vi "Read page name, size and orientation from PDF file.vi"(0 "PageSizeWithRotation":refnum<k24>, 11 "error in (no error)":errorcluster) -> (4 "PageSizeWithRotation duplicate":refnum<k24>, 8 "Pages dimensions OUT":T1={"Start at page"=-1, "Page Size"=0, "Orientation"=enum."Portrait", "widht"=0.0, "height"=0.0, "Margin left"=0.0, "Margin right"=0.0, "Margin top"=0.0, "Margin bottom"=0.0, "X0"=0.0, "X1"=612.0, "Y0"=0.0, "Y1"=792.0} {"Page Size" items=["Custom", "LETTER", "NOTE", "LEGAL", "TABLOID", "EXECUTIVE", "POSTCARD", "A0", "A1", "A2", "A3", "A4", "A5", "A6", "A7", "A8", "A9", "A10", "B0", "B1", "B2", "B3", "B4", "B5", "B6", "B7", "B8", "B9", "B10", "ARCH_E", "ARCH_D", "ARCH_C", "ARCH_B", "ARCH_A", "FLSA", "FLSE", "HALFLETTER", "_11X17", "ID_1", "ID_2", "ID_3", "LEDGER", "CROWN_QUARTO", "LARGE_CROWN_QUARTO", "DEMY_QUARTO", "ROYAL_QUARTO", "CROWN_OCTAVO", "LARGE_CROWN_OCTAVO", "DEMY_OCTAVO", "ROYAL_OCTAVO", "SMALL_PAPERBACK", "PENGUIN_SMALL_PAPERBACK", "PENGUIN_LARGE_PAPERBACK"]}, 15 "error out":errorcluster)   [LabVIEW 2019, in "Exaprom PDF.lvlib"]
doc: "Version 1.1\nDeveloped by Jean-Marc Simard\nCopyright © 2012, Exaprom Inc.\nAll rights reserved.\nLicense: BSD\n\nWith iTextSharp 4.1.6 (http://itextsharp.sourceforge.net)\nunder Mozilla Public License Version 1.1\n(http://www.mozilla.org/MPL/MPL-1.1.html)"
uses:
  C:/work/niobrara_lv/labview pdf writer fixing/DLL/itextsharp.dll
  DLL/itextsharp.dll
  Controls/Page Controls/Page dimensions.ctl
  Controls/Page Controls/Page Orientation.ctl
  Exaprom PDF.lvlib
  Controls/Page Controls/Page size.ctl
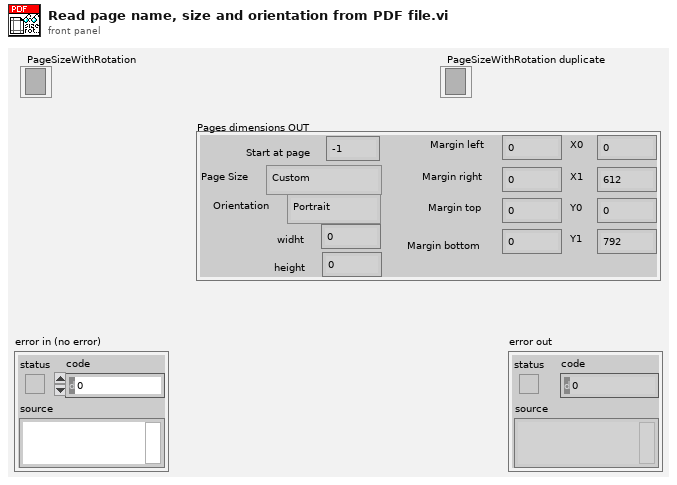
[diagram p1: front panel]
types:
  T1 = typedef "Exaprom PDF.lvlib/Page dimensions.ctl" = cluster{"Start at page":i32, "Page Size":T2, "Orientation":T3, "widht":sgl, "height":sgl, "Margin left":sgl, "Margin right":sgl, "Margin top":sgl, "Margin bottom":sgl, "X0":sgl, "X1":sgl, "Y0":sgl, "Y1":sgl}
  T2 = typedef "Exaprom PDF.lvlib/Page size.ctl" = i32
  T3 = typedef "Exaprom PDF.lvlib/Page Orientation.ctl" = enum16{"Portrait", "Landscape"}
  T4 = cluster{"Name":string, "Width":sgl, "Height":sgl}[]
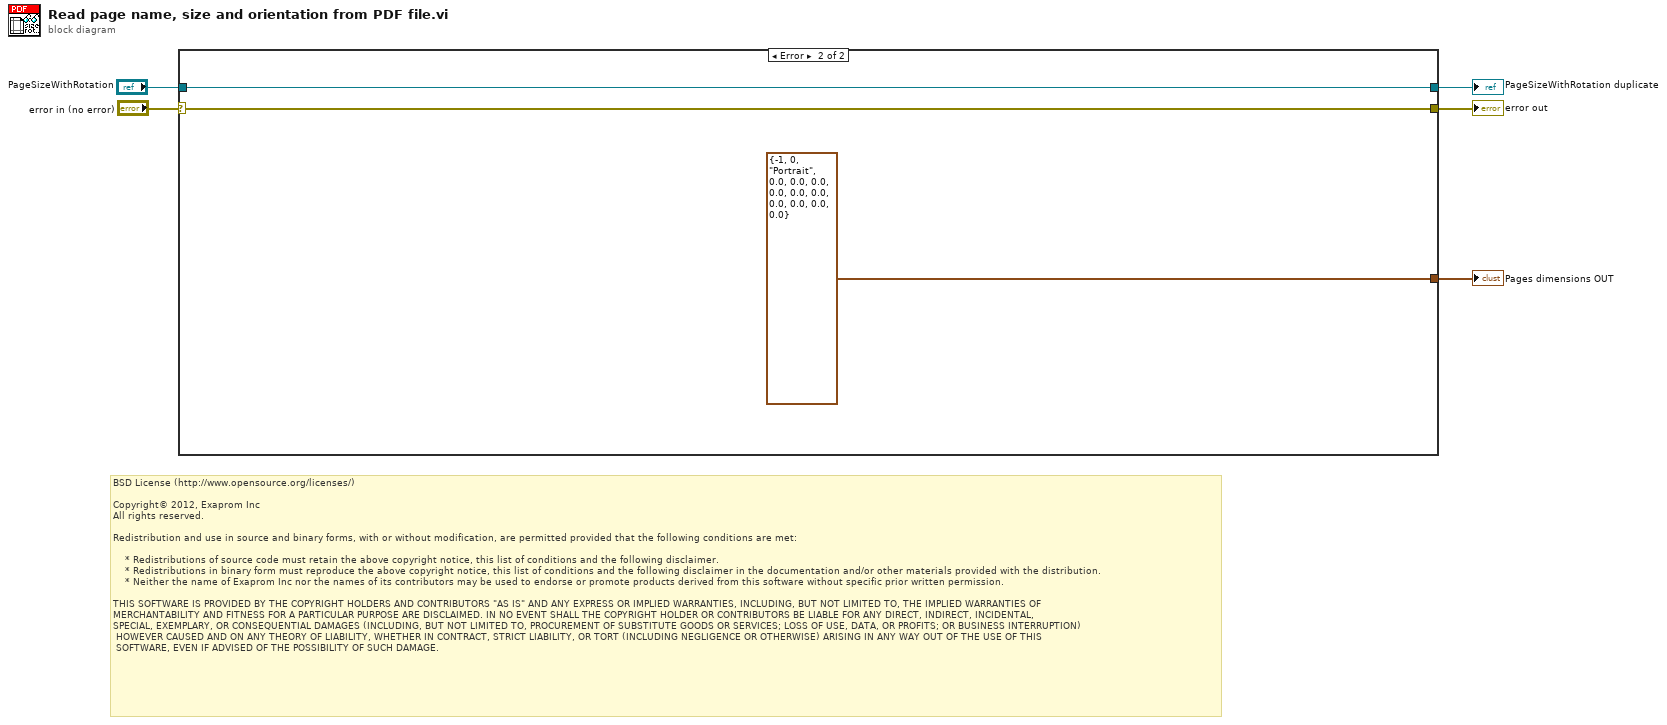
[diagram p0: block diagram]
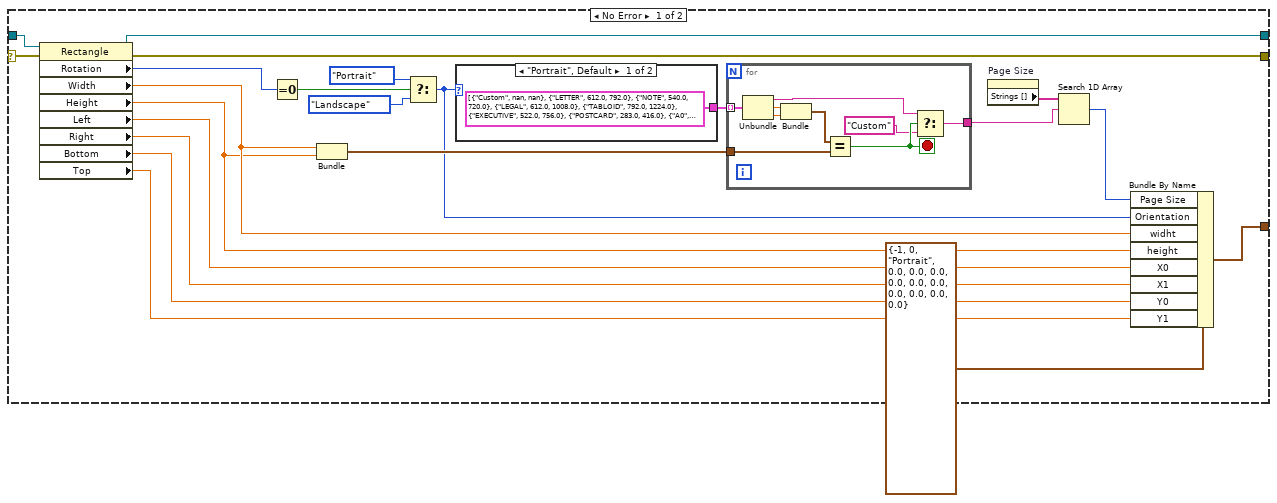
[diagram p2: hidden frame]
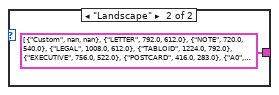
[diagram p3: hidden frame]
diagram:
  # "BSD License (http://www.opensource.org/licenses/)\n\nCopyright© 2012, Exaprom Inc\nAll rights reserved.\n\nRedistribution and use in source and binary forms, with or without modification, are permitted provided that the following conditions are met:\n\n    * Redistributions of source code must retain the above copyright notice, this list of conditions and the following disclaimer.\n    * Redistributions in binary form must reproduce the above copyright notice, this list of conditions and the following disclaimer in the documentation and/or other materials provided with the distribution.\n    * Neither the name of Exaprom Inc nor the names of its contributors may be used to endorse or promote products derived from this software without specific prior written permission.\n\nTHIS SOFTWARE IS PROVIDED BY THE COPYRIGHT HOLDERS AND CONTRIBUTORS \"AS IS\" AND ANY EXPRESS OR IMPLIED WARRANTIES, INCLUDING, BUT NOT LIMITED TO, THE IMPLIED WARRANTIES OF \nMERCHANTABILITY AND FITNESS FOR A PARTICULAR PURPOSE ARE DISCLAIMED. IN NO EVENT SHALL THE COPYRIGHT HOLDER OR CONTRIBUTORS BE LIABLE FOR ANY DIRECT, INDIRECT, INCIDENTAL,\nSPECIAL, EXEMPLARY, OR CONSEQUENTIAL DAMAGES (INCLUDING, BUT NOT LIMITED TO, PROCUREMENT OF SUBSTITUTE GOODS OR SERVICES; LOSS OF USE, DATA, OR PROFITS; OR BUSINESS INTERRUPTION)\n HOWEVER CAUSED AND ON ANY THEORY OF LIABILITY, WHETHER IN CONTRACT, STRICT LIABILITY, OR TORT (INCLUDING NEGLIGENCE OR OTHERWISE) ARISING IN ANY WAY OUT OF THE USE OF THIS\n SOFTWARE, EVEN IF ADVISED OF THE POSSIBILITY OF SUCH DAMAGE."
  n1 = case shown="Error" "error in (no error)" {
    selector: "error in (no error)" -> [w22 w41]
    tunnel: [w23 w41] -> w5
    tunnel: "PageSizeWithRotation" -> [w21 w40]
    tunnel: [w20 w40] -> w2
    tunnel: [w11 T1 {"Start at page"=-1, "Page Size"=0, "Orientation"=enum."Portrait", "widht"=0.0, "height"=0.0, "Margin left"=0.0, "Margin right"=0.0, "Margin top"=0.0, "Margin bottom"=0.0, "X0"=0.0, "X1"=0.0, "Y0"=0.0, "Y1"=0.0} ("output cluster")] -> w1
    frame No Error {
      n2 = property class="Rectangle"(reference=w21, error in=w22) -> (reference out=w20:refnum<k24>, error out=w23:errorcluster, "Rotation"=w27:i32, "Width"=w14:sgl, "Height"=w13:sgl, "Left"=w9:sgl, "Right"=w8:sgl, "Bottom"=w7:sgl, "Top"=w6:sgl)
      n3 = Equal To 0?(x=w27) -> (x = 0?=w26:bool)
      n4 = Bundle("Width"=w14, "Height"=w13) -> (w18:cluster{"Width":sgl, "Height":sgl})  [unwired: 1 in]
      n5 = Select(t=Page_Orientation."Portrait" ("Orientation"), s=w26, f=Page_Orientation."Landscape" ("Orientation")) -> (s? t:f=w15:T3)
      n6 = case shown="\"Portrait\", Default" w15 {
        tunnel: [T4 [{"Name"="Custom", "Width"=nan, "Height"=nan}, {"Name"="LETTER", "Width"=612.0, "Height"=792.0}, {"Name"="NOTE", "Width"=540.0, "Height"=720.0}, {"Name"="LEGAL", "Width"=612.0, "Height"=1008.0}, {"Name"="TABLOID", "Width"=792.0, "Height"=1224.0}, {"Name"="EXECUTIVE", "Width"=522.0, "Height"=756.0}, {"Name"="POSTCARD", "Width"=283.0, "Height"=416.0}, {"Name"="A0", "Width"=2384.0, "Height"=3370.0}, {"Name"="A1", "Width"=1684.0, "Height"=2384.0}, {"Name"="A2", "Width"=1191.0, "Height"=1684.0}, {"Name"="A3", "Width"=842.0, "Height"=1191.0}, {"Name"="A4", "Width"=595.0, "Height"=842.0}, {"Name"="A5", "Width"=420.0, "Height"=595.0}, {"Name"="A6", "Width"=297.0, "Height"=420.0}, {"Name"="A7", "Width"=210.0, "Height"=297.0}, {"Name"="A8", "Width"=148.0, "Height"=210.0}, {"Name"="A9", "Width"=105.0, "Height"=148.0}, {"Name"="A10", "Width"=73.0, "Height"=105.0}, {"Name"="B0", "Width"=2834.0, "Height"=4008.0}, {"Name"="B1", "Width"=2004.0, "Height"=2834.0}, {"Name"="B2", "Width"=1417.0, "Height"=2004.0}, {"Name"="B3", "Width"=1000.0, "Height"=1417.0}, {"Name"="B4", "Width"=708.0, "Height"=1000.0}, {"Name"="B5", "Width"=498.0, "Height"=708.0}, {"Name"="B6", "Width"=354.0, "Height"=498.0}, {"Name"="B7", "Width"=249.0, "Height"=354.0}, {"Name"="B8", "Width"=175.0, "Height"=249.0}, {"Name"="B9", "Width"=124.0, "Height"=175.0}, {"Name"="B10", "Width"=87.0, "Height"=124.0}, {"Name"="ARCH_E", "Width"=2592.0, "Height"=3456.0}, {"Name"="ARCH_D", "Width"=1728.0, "Height"=2592.0}, {"Name"="ARCH_C", "Width"=1296.0, "Height"=1728.0}, {"Name"="ARCH_B", "Width"=864.0, "Height"=1296.0}, {"Name"="ARCH_A", "Width"=648.0, "Height"=864.0}, {"Name"="FLSA", "Width"=612.0, "Height"=936.0}, {"Name"="FLSE", "Width"=648.0, "Height"=936.0}, {"Name"="HALFLETTER", "Width"=396.0, "Height"=612.0}, {"Name"="_11X17", "Width"=792.0, "Height"=1224.0}, {"Name"="ID_1", "Width"=242.65, "Height"=153.0}, {"Name"="ID_2", "Width"=297.0, "Height"=210.0}, {"Name"="ID_3", "Width"=354.0, "Height"=249.0}, {"Name"="LEDGER", "Width"=1224.0, "Height"=792.0}, {"Name"="CROWN_QUARTO", "Width"=535.0, "Height"=697.0}, {"Name"="LARGE_CROWN_QUARTO", "Width"=569.0, "Height"=731.0}, {"Name"="DEMY_QUARTO", "Width"=620.0, "Height"=782.0}, {"Name"="ROYAL_QUARTO", "Width"=671.0, "Height"=884.0}, {"Name"="CROWN_OCTAVO", "Width"=348.0, "Height"=527.0}, {"Name"="LARGE_CROWN_OCTAVO", "Width"=365.0, "Height"=561.0}, {"Name"="DEMY_OCTAVO", "Width"=391.0, "Height"=612.0}, {"Name"="ROYAL_OCTAVO", "Width"=442.0, "Height"=663.0}, {"Name"="SMALL_PAPERBACK", "Width"=314.0, "Height"=504.0}, {"Name"="PENGUIN_SMALL_PAPERBACK", "Width"=314.0, "Height"=513.0}, {"Name"="PENGUIN_LARGE_PAPERBACK", "Width"=365.0, "Height"=561.0}] ("Portrait") T4 [{"Name"="Custom", "Width"=nan, "Height"=nan}, {"Name"="LETTER", "Width"=792.0, "Height"=612.0}, {"Name"="NOTE", "Width"=720.0, "Height"=540.0}, {"Name"="LEGAL", "Width"=1008.0, "Height"=612.0}, {"Name"="TABLOID", "Width"=1224.0, "Height"=792.0}, {"Name"="EXECUTIVE", "Width"=756.0, "Height"=522.0}, {"Name"="POSTCARD", "Width"=416.0, "Height"=283.0}, {"Name"="A0", "Width"=3370.0, "Height"=2384.0}, {"Name"="A1", "Width"=2384.0, "Height"=1684.0}, {"Name"="A2", "Width"=1684.0, "Height"=1191.0}, {"Name"="A3", "Width"=1191.0, "Height"=842.0}, {"Name"="A4", "Width"=842.0, "Height"=595.0}, {"Name"="A5", "Width"=595.0, "Height"=420.0}, {"Name"="A6", "Width"=420.0, "Height"=297.0}, {"Name"="A7", "Width"=297.0, "Height"=210.0}, {"Name"="A8", "Width"=210.0, "Height"=148.0}, {"Name"="A9", "Width"=148.0, "Height"=105.0}, {"Name"="A10", "Width"=105.0, "Height"=73.0}, {"Name"="B0", "Width"=4008.0, "Height"=2834.0}, {"Name"="B1", "Width"=2834.0, "Height"=2004.0}, {"Name"="B2", "Width"=2004.0, "Height"=1417.0}, {"Name"="B3", "Width"=1417.0, "Height"=1000.0}, {"Name"="B4", "Width"=1000.0, "Height"=708.0}, {"Name"="B5", "Width"=708.0, "Height"=498.0}, {"Name"="B6", "Width"=498.0, "Height"=354.0}, {"Name"="B7", "Width"=354.0, "Height"=249.0}, {"Name"="B8", "Width"=249.0, "Height"=175.0}, {"Name"="B9", "Width"=175.0, "Height"=124.0}, {"Name"="B10", "Width"=124.0, "Height"=87.0}, {"Name"="ARCH_E", "Width"=3456.0, "Height"=2592.0}, {"Name"="ARCH_D", "Width"=2592.0, "Height"=1728.0}, {"Name"="ARCH_C", "Width"=1728.0, "Height"=1296.0}, {"Name"="ARCH_B", "Width"=1296.0, "Height"=864.0}, {"Name"="ARCH_A", "Width"=864.0, "Height"=648.0}, {"Name"="FLSA", "Width"=936.0, "Height"=612.0}, {"Name"="FLSE", "Width"=936.0, "Height"=648.0}, {"Name"="HALFLETTER", "Width"=612.0, "Height"=396.0}, {"Name"="_11X17", "Width"=1224.0, "Height"=792.0}, {"Name"="ID_1", "Width"=153.0, "Height"=242.65}, {"Name"="ID_2", "Width"=210.0, "Height"=297.0}, {"Name"="ID_3", "Width"=249.0, "Height"=354.0}, {"Name"="LEDGER", "Width"=792.0, "Height"=1224.0}, {"Name"="CROWN_QUARTO", "Width"=697.0, "Height"=535.0}, {"Name"="LARGE_CROWN_QUARTO", "Width"=731.0, "Height"=569.0}, {"Name"="DEMY_QUARTO", "Width"=782.0, "Height"=620.0}, {"Name"="ROYAL_QUARTO", "Width"=884.0, "Height"=671.0}, {"Name"="CROWN_OCTAVO", "Width"=527.0, "Height"=348.0}, {"Name"="LARGE_CROWN_OCTAVO", "Width"=561.0, "Height"=365.0}, {"Name"="DEMY_OCTAVO", "Width"=612.0, "Height"=391.0}, {"Name"="ROYAL_OCTAVO", "Width"=663.0, "Height"=442.0}, {"Name"="SMALL_PAPERBACK", "Width"=504.0, "Height"=314.0}, {"Name"="PENGUIN_SMALL_PAPERBACK", "Width"=513.0, "Height"=314.0}, {"Name"="PENGUIN_LARGE_PAPERBACK", "Width"=561.0, "Height"=365.0}] ("Landscape")] -> w19
        frame "Portrait", Default {
        }
        frame "Landscape" {
        }
      }
      n7 = for {
        tunnel: w19 -> [w36] mode=indexing
        tunnel: w18 -> [w28]
        tunnel: [w29] -> w17
        stop <- w32 stop-if-true
        n8 = Unbundle(w36) -> ("Name"=w30:string, "Width"=w35:sgl, "Height"=w34:sgl)
        n9 = Bundle("Width"=w35, "Height"=w34) -> (w33:cluster{"Width":sgl, "Height":sgl})  [unwired: 1 in]
        n10 = Equal?(x=w33, y=w28) -> (x = y?=w32:bool)
        n11 = Select(t=w30, s=w32, f="Custom") -> (s? t:f=w29:string)
      }
      n12 = property on="Page Size" class="Ring (strict)"() -> ("Strings []"=w10:string[])  [unwired: 2 in, 2 out]
      n13 = Search 1D Array(1D array=w10, element=w17) -> (index of element=w16:i32)  [unwired: 1 in]
      n14 = Bundle By Name(cluster=T1 {"Start at page"=-1, "Page Size"=0, "Orientation"=enum."Portrait", "widht"=0.0, "height"=0.0, "Margin left"=0.0, "Margin right"=0.0, "Margin top"=0.0, "Margin bottom"=0.0, "X0"=0.0, "X1"=0.0, "Y0"=0.0, "Y1"=0.0} ("output cluster"), "Page Size"=w16, "Orientation"=w15, "widht"=w14, "height"=w13, "X0"=w9, "X1"=w8, "Y0"=w7, "Y1"=w6) -> (w11:T1)
    }
    frame Error {
    }
  }
  "error out" <- w5
  "PageSizeWithRotation duplicate" <- w2
  "Pages dimensions OUT" <- w1
